vi "writepulseblaster.vi"(8 "error in (no error)":errorcluster, 10 "Instructions":T1(array[cluster])=[{"Instruct Data"=0, "Op Code"=0, "Flags"=[TRUE, FALSE, FALSE, FALSE, FALSE, FALSE, FALSE, FALSE, FALSE, FALSE, FALSE, FALSE, FALSE, FALSE, FALSE, FALSE, FALSE, FALSE, FALSE, FALSE, FALSE, FALSE, FALSE, FALSE], "Comments"="", "Time (s)"=0.1}, {"Instruct Data"=0, "Op Code"=0, "Flags"=[FALSE, FALSE, FALSE, FALSE, FALSE, FALSE, FALSE, FALSE, FALSE, FALSE, FALSE, FALSE, FALSE, FALSE, FALSE, FALSE, FALSE, FALSE, FALSE, FALSE, FALSE, FALSE, FALSE, FALSE], "Comments"="", "Time (s)"=0.1}, {"Instruct Data"=0, "Op Code"=0, "Flags"=[TRUE, FALSE, FALSE, FALSE, FALSE, FALSE, FALSE, FALSE, FALSE, FALSE, FALSE, FALSE, FALSE, FALSE, FALSE, FALSE, FALSE, FALSE, FALSE, FALSE, FALSE, FALSE, FALSE, FALSE], "Comments"="", "Time (s)"=0.1}, {"Instruct Data"=0, "Op Code"=6, "Flags"=[FALSE, FALSE, FALSE, FALSE, FALSE, FALSE, FALSE, FALSE, FALSE, FALSE, FALSE, FALSE, FALSE, FALSE, FALSE, FALSE, FALSE, FALSE, FALSE, FALSE, FALSE, FALSE, FALSE, FALSE], "Comments"="", "Time (s)"=0.1}] {"Time (s)" format="%.3p"; "Op Code" items=["Continue", "Stop", "Loop", "End Loop", "JSR", "RTS", "Branch", "Long Delay", "Wait"]}) -> (0 "error out":errorcluster)   [LabVIEW 2013]
panel:
  # "1"
  # "2"
  # "3"
  # "4"
  # "5"
  # "6"
  # "7"
  # "8"
  # "9"
  # "10"
  # "11"
  # "12"
  # "13"
  # "14"
  # "15"
  # "16"
  # "17"
  # "18"
  # "19"
  # "20"
  # "21"
  # "22"
  # "23"
  # "24"
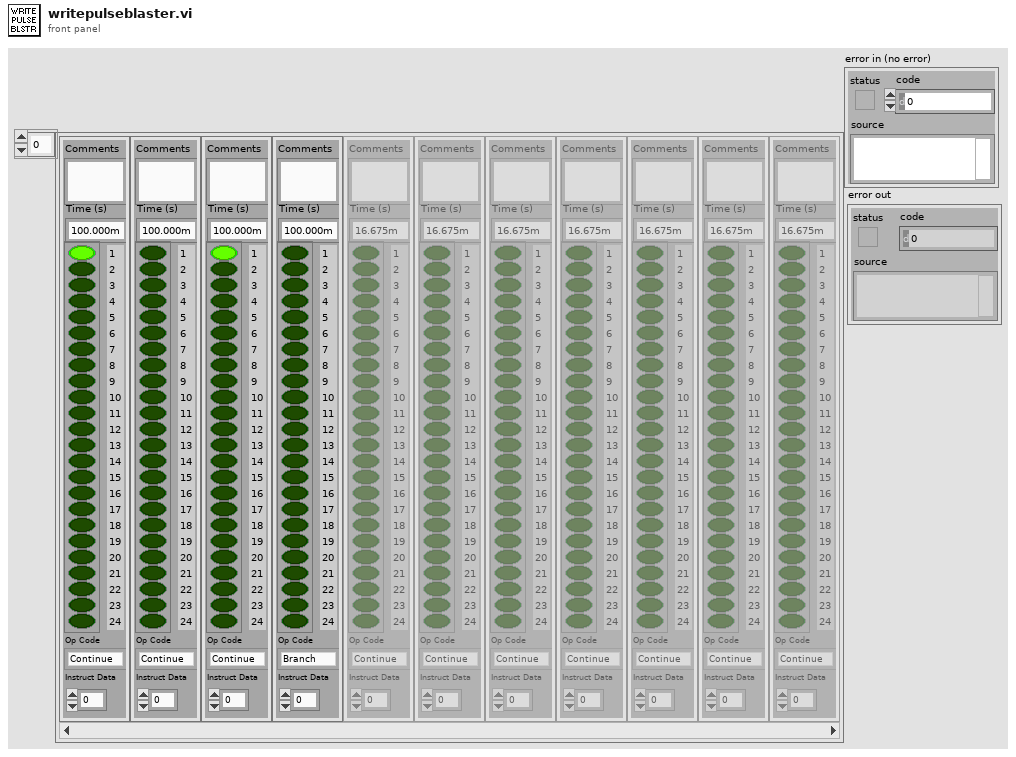
[diagram p1: front panel]
types:
  T1 = cluster{"Instruct Data":i32, "Op Code":i32, "Flags":bool[], "Comments":string, "Time (s)":dbl}[]
  T2 = enum16{"Pulse Program", "Frequency Registers", "TX Phase Registers", "RX Phase Registers"}
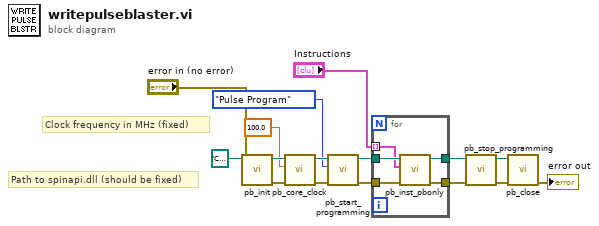
[diagram p0: block diagram]
diagram:
  # "Path to spinapi.dll (should be fixed)"
  # "Clock frequency in MHz (fixed)"
  n1 = call "pb_init.vi"("error in (no error)"="error in (no error)", "path in"=path "C:/SpinCore/SpinAPI/lib32/spinapi.dll") -> ("error out"=w10:errorcluster, "path out"=w15:path)  [unwired: 2 in, 6 out]
  n2 = call "pb_core_clock.vi"("error in (no error)"=w10, "clock_freq (MHz)"=100.0, "path in"=w15) -> ("error out"=w9:errorcluster, "path out"=w14:path)  [unwired: 7 in]
  n3 = call "pb_start_programming.vi"("error in (no error)"=w9, "Device"=T2."Pulse Program", "path in"=w14) -> ("error out"=w8:errorcluster, "path out"=w13:path)  [unwired: 1 in, 6 out]
  n4 = for {
    tunnel: w13 -> [w21]
    tunnel: [w20] -> w12
    tunnel: w8 -> [w19]
    tunnel: [w18] -> w7
    tunnel: "Instructions" -> [w17] mode=indexing
    n5 = call "pb_inst_pbonly.vi"("error in (no error)"=w19, "PB Instruction"=w17, "path in"=w21) -> ("error out"=w18:errorcluster, "path out"=w20:path)  [unwired: 2 in, 5 out]
  }
  n6 = call "pb_stop_programming.vi"("error in (no error)"=w7, "path in"=w12) -> ("error out"=w6:errorcluster, "path out"=w11:path)  [unwired: 1 in, 7 out]
  n7 = call "pb_close.vi"("error in (no error)"=w6, "path in"=w11) -> ("error out"=→"error out":errorcluster)  [unwired: 9 out]
